vi "Choreo_TrajectoryCacheDifferential_LoadTrajectory.vi"(11 "TrajectoryName":string) -> (0 "error out":errorcluster, 3 "ChoreoTrajectoryDifferential":T1)   [LabVIEW 2019, in "ChoreoLib.lvlib"]
doc: "Load a Differential trajectory from the memory cache. If the trajectory doesn't exist in the cache is is read from the file system default choreo directory. Choreolib expects .traj files to be placed in /deploy/choreo/<trajectoryName>.traj.\n\nInputs: \n - TrajectoryName - string - The name of the trajectory. This should NOT have a .traj file extension.\n - ErrorIn - cluster - standard error cluster\n\nOutputs:\n - ChoreoDifferentialTrajectory - cluster - The trajectory obtained from the cache or from a file.\n - InCache - boolean - TRUE if the trajectory was found in the cache.\n - ErrorOut - cluster - Error cluster"
uses:
  ChoreoLib.lvlib
  TypeDef/ChoreoTrajectoryDifferential.ctl
  TypeDef/ChoreoDifferentialSample.ctl
  TypeDef/ChoreoEventMarker.ctl
  Choreo_Choreo_Globals.vi
panel:
  out "InCache":bool
  in  "error in (no error)":errorcluster
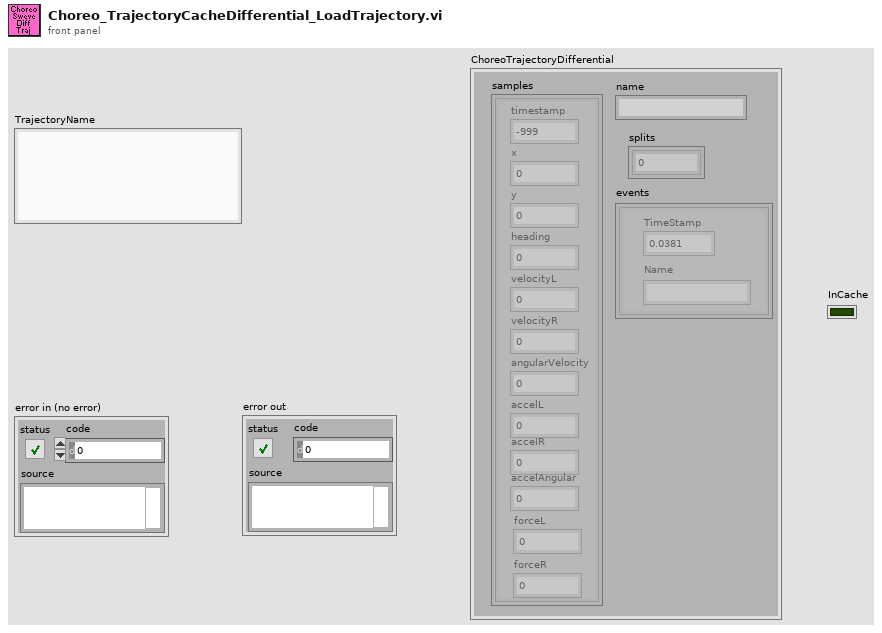
[diagram p1: front panel]
types:
  T1 = typedef "ChoreoLib.lvlib/ChoreoTrajectoryDifferential.ctl" = cluster{"name":string, "samples":T2[], "splits":i32[], "events":T3[]}
  T2 = typedef "ChoreoLib.lvlib/ChoreoDifferentialSample.ctl" = cluster{"timestamp":dbl, "x":dbl, "y":dbl, "heading":dbl, "velocityL":dbl, "velocityR":dbl, "angularVelocity":dbl, "accelL":dbl, "accelR":dbl, "accelAngular":dbl, "forceL":dbl, "forceR":dbl}
  T3 = typedef "ChoreoLib.lvlib/ChoreoEventMarker.ctl" = cluster{"TimeStamp":dbl, "Name":string}
  T4 = typedef "ChoreoLib.lvlib/ChoreoTrajectoryCacheDifferential.ctl" = map{string, T1}
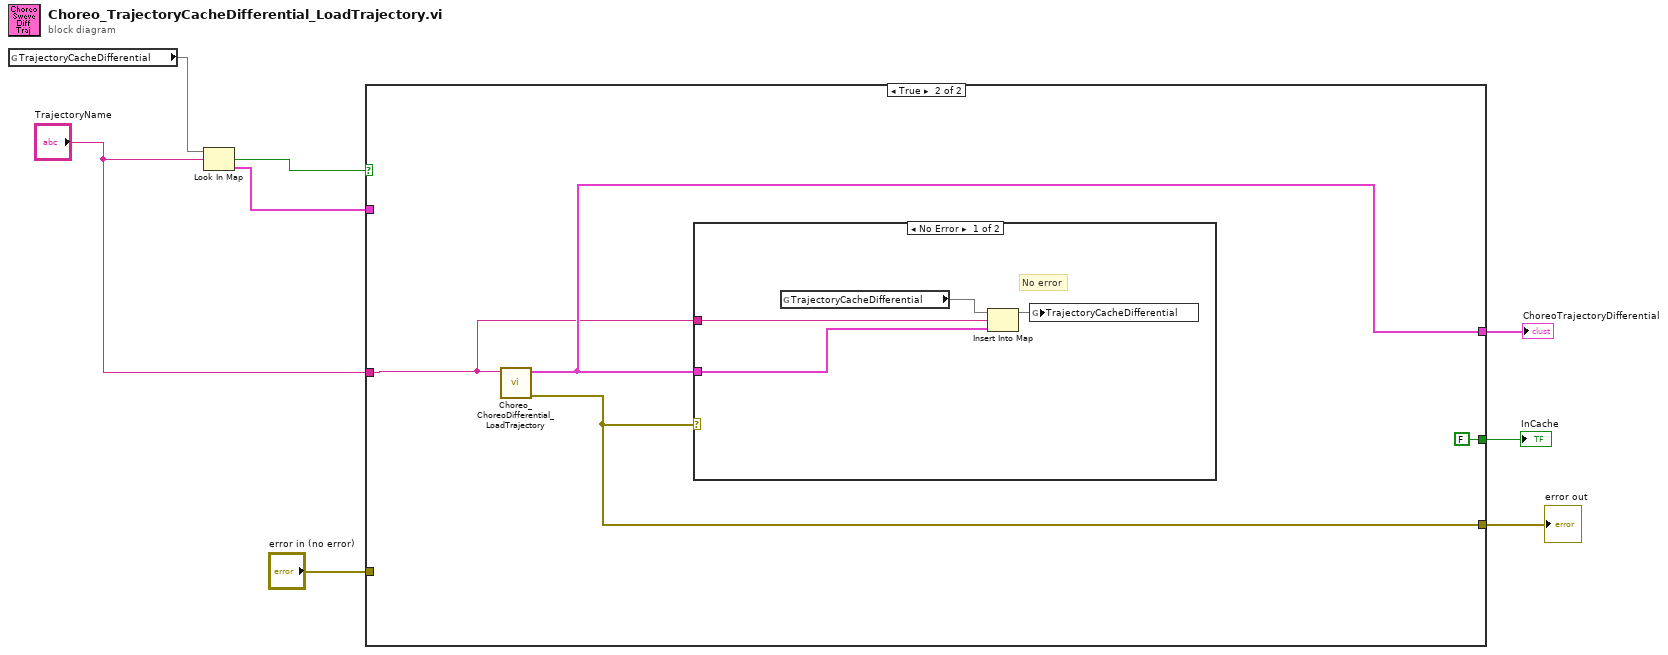
[diagram p0: block diagram]
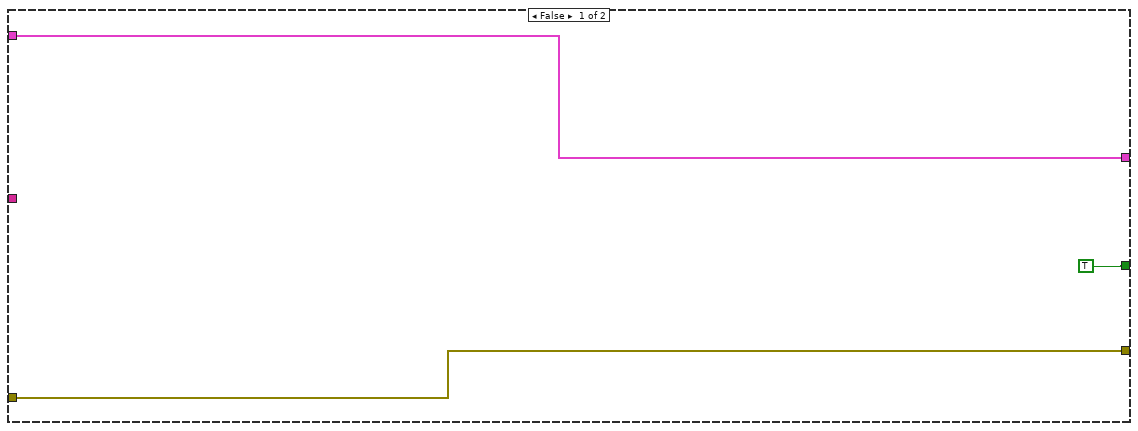
[diagram p2: hidden frame]
diagram:
  n1 = global read "Choreo_Choreo_Globals.vi" "TrajectoryCacheDifferential"() -> (w5:T4)
  n2 = Look In Map(map=w5, key="TrajectoryName") -> (key not found?=w3:bool, value=w2:T1)  [unwired: 1 in]
  n3 = case shown="True" w3 {
    tunnel: "error in (no error)" -> [w10 _]
    tunnel: [w10 w15] -> w7
    tunnel: [w11 w14] -> w6
    tunnel: "TrajectoryName" -> [_ w13]
    tunnel: w2 -> [w11 _]
    tunnel: [TRUE FALSE] -> w1
    frame False {
    }
    frame True {
      n4 = call "Choreo_ChoreoDifferential_LoadTrajectory.vi"("FileName"=w13) -> ("error out"=w15:errorcluster, "ChoreoTrajectoryDifferential"=w14:T1)  [unwired: 8 in, 1 out]
      n5 = case shown="No Error" w15 {
        tunnel: w14 -> [w17 _]
        tunnel: w13 -> [w16 _]
        frame No Error {
          # "No error"
          n6 = global read "Choreo_Choreo_Globals.vi" "TrajectoryCacheDifferential"() -> (w19:T4)
          n7 = Insert Into Map(map in=w19, key=w16, value=w17) -> (map out=w18:T4)  [unwired: 2 out]
          n8 = global write "Choreo_Choreo_Globals.vi" "TrajectoryCacheDifferential"(w18) -> ()
        }
        frame Error {
        }
      }
    }
  }
  "error out" <- w7
  "ChoreoTrajectoryDifferential" <- w6
  "InCache" <- w1
